vi "BuildResultFilename.vi"(0 "S/N":string, 5 "TEMP":string="25C", 6 "UseTimeStamp(T)":bool, 7 "Directory":string="C:\\IdtATE\\Results\\F1200_SParameter\\IOR\\", 8 "Voltage":string, 9 "Chip Type":string, 10 "Test":string, 11 "Gainctl":string) -> (4 "File Name Out":string)   [LabVIEW 2018]
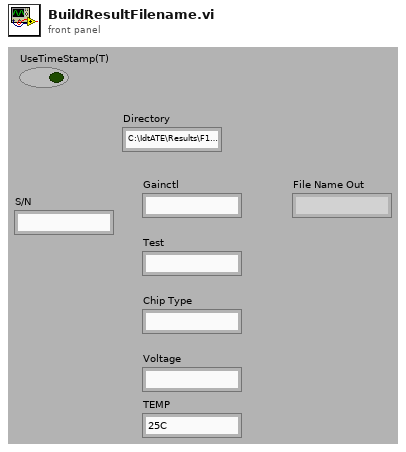
[diagram p1: front panel]
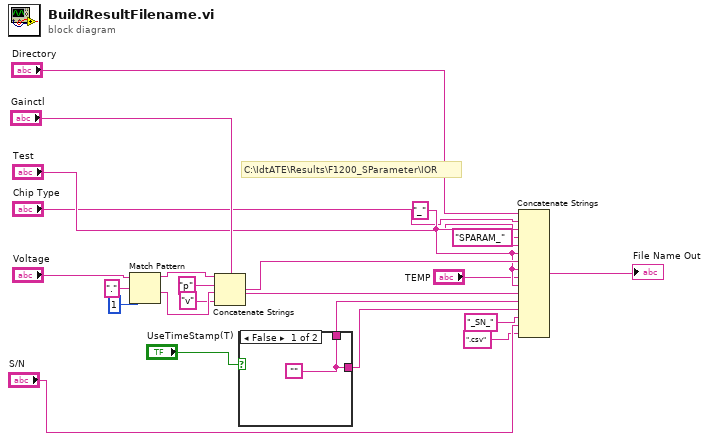
[diagram p0: block diagram]
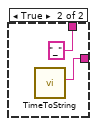
[diagram p2: hidden frame]
diagram:
  w12 = "_" ("string")
  # "C:\\IdtATE\\Results\\F1200_SParameter\\IOR"
  n1 = Match Pattern(string="Voltage", regular expression=".", offset (0)=1) -> (before substring=w22:string, after substring=w18:string)  [unwired: 2 out]
  n2 = Concatenate Strings(w22, "p" ("string"), w18, "v" ("string")) -> (w20:string)
  n3 = case shown="False" "UseTimeStamp(T)" {
    tunnel: [w23 w25] -> w13
    tunnel: [w23 "_" ("string")] -> w4
    frame False {
      w23 = ""
    }
    frame True {
      n4 = call "TimeToString.vi"() -> ("F-format string"=w25:string)  [unwired: 11 in]
    }
  }
  n5 = Concatenate Strings("Directory", "Chip Type", w12, "SPARAM_" ("string"), "Test", w12, w20, w12, "TEMP", w12, "Gainctl", w4, w13, "_SN_" ("string"), "S/N", ".csv" ("string")) -> (→"File Name Out":string)
